vi "test Write Element of TagDistanceArray.vi"(8 "error in (no error)":errorcluster, 11 "TestCase in":refnum<class "AnchorTests.lvclass">) -> (0 "error out":errorcluster, 3 "TestCase out":refnum<class "AnchorTests.lvclass">)   [LabVIEW 2014, in "AnchorTests.lvclass"]
uses:
  AnchorTests.lvclass
  SPLAT/Anchor/Anchor.lvclass
  <vilib>/addons/_JKI Toolkits/VI Tester/TestCase.llb/TestCase.lvclass
  SPLAT/Tag.lvclass
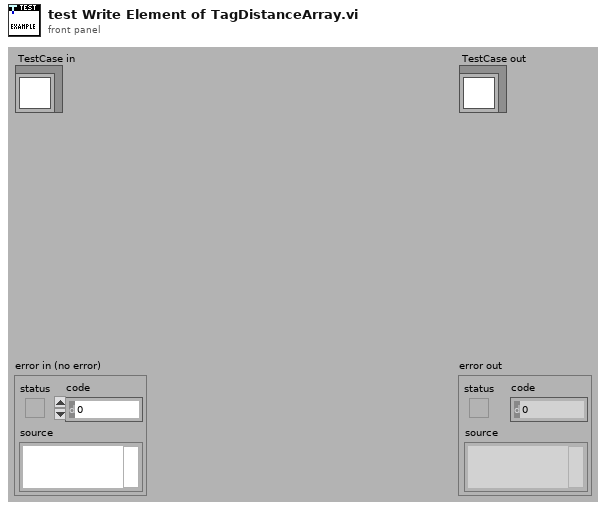
[diagram p1: front panel]
types:
  T1 = cluster{"Tag Out":refnum<class "Tag.lvclass">, "Distance":dbl}
  T2 = cluster{"Tag.lvclass":refnum<class "Tag.lvclass">, "Distance":dbl}[]
  T3 = cluster{"Tag.lvclass":refnum<class "Tag.lvclass">, "Distance":dbl}
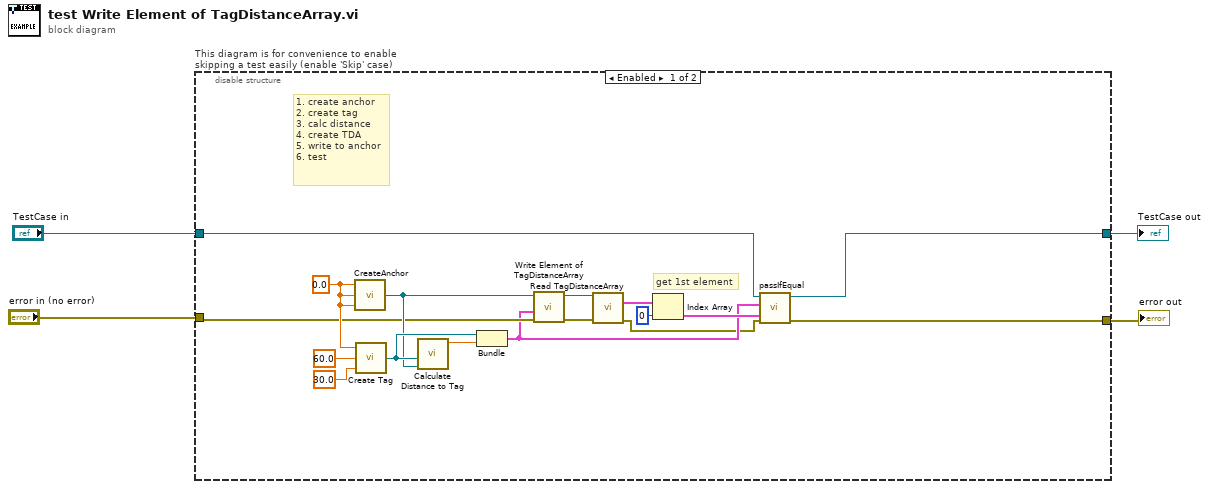
[diagram p0: block diagram]
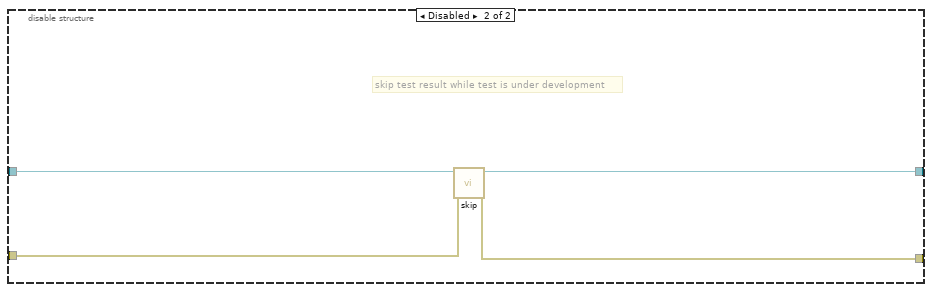
[diagram p2: hidden frame]
diagram:
  n1 = disable-structure "This diagram is for convenience to enable skipping a test easily (enable 'Skip' case)" shown="Enabled" {
    disable-tunnel: "TestCase in" -> [w8 w25]
    disable-tunnel: [w5 w23] -> w1
    disable-tunnel: [w6 w24] -> w3
    disable-tunnel: "error in (no error)" -> [w13 w22]
    frame Enabled {
      w21 = 0.0 ("Anchor ID")
      # "get 1st element"
      # "1. create anchor\n2. create tag\n3. calc distance\n4. create TDA\n5. write to anchor\n6. test"
      n2 = call "CreateAnchor.vi"("Anchor Y"=w21, "Anchor X"=w21, "Anchor ID"=w21) -> ("Anchor Out"=w16:refnum<class "Anchor.lvclass">)
      n3 = call "Create Tag.vi"("TagY"=30.0, "TagX"=60.0, "TagID"=w21) -> ("Tag Out"=w18:refnum<class "Tag.lvclass">)
      n4 = call "Calculate Distance to Tag.vi"("Anchor.lvclass In"=w16, "Tag.lvclass"=w18) -> ("Distance"=w17:dbl)  [unwired: 8 in, 1 out]
      n5 = Bundle("Tag Out"=w18, "Distance"=w17) -> (w9:T1)  [unwired: 1 in]
      n6 = call-dynamic "Write Element of TagDistanceArray.vi"("error in (no error)"=w13, "TagDistance"=w9, "Anchor in"=w16) -> ("error out"=w15:errorcluster, "Anchor out"=w14:refnum<class "Anchor.lvclass">)  [unwired: 7 in]
      n7 = call-dynamic "Read TagDistanceArray.vi"("error in (no error)"=w15, "Anchor in"=w14) -> ("error out"=w7:errorcluster, "TagDistanceArray"=w12:T2)  [unwired: 7 in, 1 out]
      n8 = Index Array(array=w12, index=0) -> (element=w10:T3)
      n9 = call-dynamic "passIfEqual.vi"("error in (no error)"=w7, "y"=w10, "x"=w9, "TestCase in"=w8) -> ("error out"=w6:errorcluster, "TestCase out"=w5:refnum<class "AnchorTests.lvclass">)  [unwired: 6 in]
    }
    frame Disabled {
      # "skip test result while test is under development"
      n10 = call <vilib>:"skip.vi"("error in (no error)"=w22, "TestCase in"=w25) -> ("error out"=w24:errorcluster, "TestCase out"=w23:refnum<class "AnchorTests.lvclass">)  [unwired: 8 in]
    }
  }
  "error out" <- w3
  "TestCase out" <- w1
